vi "createTimeTagger.vi"(8 "error in (no error)":errorcluster, 10 "resolution":i32(ring) items=["Standard", "HighResA", "HighResB", "HighResC"], 11 "serial":string) -> (0 "error out":errorcluster, 3 "TimeTagger ref out":refnum<k24>)   [LabVIEW 2014]
doc: "Create Time Tagger object for the device identified by the serial number.\nWhen \"serial\" is an emtpty string a first detected Time Tagger device will be used."
uses:
  SwabianInstruments.TimeTagger
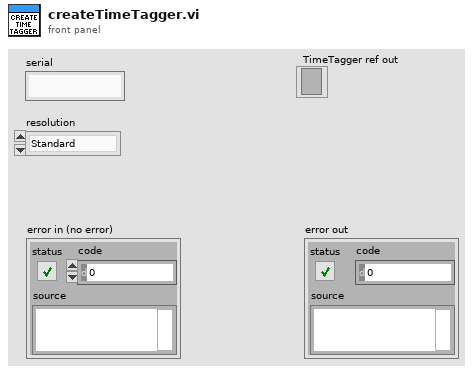
[diagram p1: front panel]
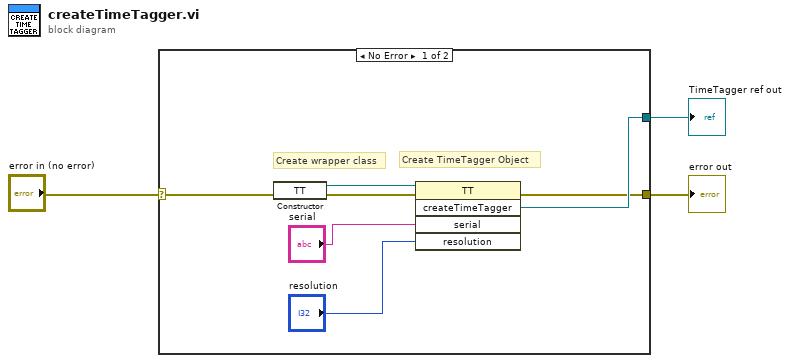
[diagram p0: block diagram]
diagram:
  n1 = case shown="No Error" "error in (no error)" {
    selector: "error in (no error)" -> [w8 w11]
    tunnel: [w7 _] -> w3
    tunnel: [w6 w11] -> w2
    frame No Error {
      # "Create wrapper class"
      # "Create TimeTagger Object"
      n2 = constructor class="TT" ("Constructor Node")(error in=w8) -> (reference out=w9:refnum<k24>, error out=w10:errorcluster)  [unwired: 2 in, 1 out]
      n3 = invoke class="TT" method="createTimeTagger"(reference=w9, error in=w10, "serial"="serial", "resolution"="resolution") -> (error out=w6:errorcluster, "createTimeTagger"=w7:refnum<k24>)  [unwired: 1 in, 3 out]
    }
    frame Error {
    }
  }
  "TimeTagger ref out" <- w3
  "error out" <- w2
